vi "RT Main v0.8.vi"() -> ()   [LabVIEW 2017]
uses:
  support/Controls/All Inputs.ctl
  support/Controls/Index Details.ctl
  Controls/Auto Delays.ctl
  Global Variables/RT GV.vi
  <vilib>/Utility/error.llb/Error Cluster From Error Code.vi
  <vilib>/rvi/errors/niLvFpgaAdjustHostInterfaceError.vi
  Global Variables/FPGA GV.vi
  Global Variables/Network Globals.vi
  support/Message Queue/Enqueue Message (Single).vi
  <vilib>/FPGAPlugInAG/Dynamic/niLvFpga_Close_Dynamic.vi
  <vilib>/rvi/interface/nirviReadWriteControl/nirviReadWriteControl.xnode
  Controls/FPGA Ref.ctl
  <vilib>/rvi/interface/nirviCloseFPGA/nirviCloseFPGA.xnode
  support/Message Queue/Message Queue.lvlib
  NiFpgaLv.dll
  <vilib>/rvi/interface/Simulation/niFpgaSimulationCallBeginRW.vi
panel:
  out "BF Delays":u32[](array[numeric])=[1000, 1000]
  in  "Stop Button 3":bool
  in  "Stop Button 2":bool
  out "Agitator Delays":u32[](array[numeric])=[400, 5000]
  out "error out":errorcluster
  out "Wrong Message":string
  in  "Stop Button":bool
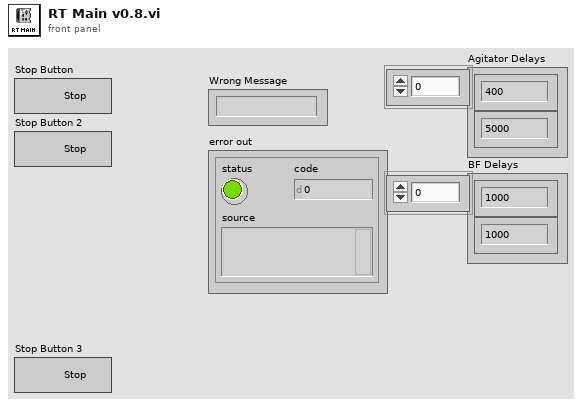
[diagram p1: front panel]
types:
  T1 = typedef "FPGA Ref.ctl" = refnum<k20>
  T2 = cluster{"TL_Red":bool, "TL_Orange":bool, "TL_Green":bool, "TL_Buzzer":bool, "SOL_Index_Rotary_CW":bool, "SOL_Index_CNVR_Rotary_CCW":bool, "SOL_Index_CNVR_Stopper_Rear":bool, "SOL_Index_CNVR_Output _Separator _Rear":bool, "Bowl  Feeder_ ON":bool, "Pump_CNVR_Motor _ON":bool, "SOL_Gating_CYL_Rear":bool, "SOL_Tube_Feed_Agitatator":bool, "SOL_Tube_Feed_Gating_CYL":bool, "SOL_Insertion _CYL":bool, "SOL_Insertion_Clamp_CYL":bool, "SOL_Cutting_CYL":bool, "SOL_Cutting_Clamp_CYL":bool, "SOL_Insertion_Air_Nozzle":bool, "SOL_Measurement_CYL":bool, "SOL_Measure_Clamp_CYL":bool, "SOL_Rejection CYL_1":bool, "SOL_Rejection CYL_2":bool, "SOL_Rejection CYL_3":bool, "SOL_Rejection CYL_4":bool, "DO1.24":bool, "DO1.25":bool, "DO1.26":bool, "DO1.27":bool, "DO1.28":bool, "DO1.29":bool, "DO1.30":bool, "DO1.31":bool}
  T3 = typedef "All Inputs.ctl" = cluster{"DI 1":cluster{"Machine_ON":bool, "E_stop ":bool, "SW_Pressure":bool, "SW_Start ":bool, "SW_Reset":bool, "SW_Stop":bool, "SW_Door":bool, "RS_Index_Rotary_CW":bool, "RS_Index_Rotary_CCW":bool, "RS_Index_Stopper _Rear":bool, "RS_Index_Output_Separator_Rear":bool, "PES_Index_Pallet_Sensor":bool, "PES_Index_Output_Part Sensor":bool, "ICS_BF_Low_Level_1":bool, "ICS_BF_Low_Level_2":bool, "ICS_BF_Pump_CNVR_Full_1":bool, "ICS_BF_Pump_CNVR_Full_2":bool, "ICS_BF_Pump_CNVR_Full_3":bool, "ICS_BF_Pump_CNVR_Full_4":bool, "PES_PC_Pump Presence_1":bool, "PES_PC_Pump Presence_2":bool, "PES_PC_Pump Presence_3":bool, "PES_PC_Pump Presence_4":bool, "RS_PC_Gating_Front":bool, "PES_Pump_Interference":bool, "PES_TF_Low_Level":bool, "PES_Tube Presence_1":bool, "PES_Tube Presence_2":bool, "PES_Tube Presence_3":bool, "PES_Tube Presence_4":bool, "DI1.30":bool, "DI1.31":bool}, "DI 2":cluster{"RS_Agitatator_1_Rear ":bool, "RS_Agitatator_2_Rear ":bool, "RS_TF_Gating CYL_Rear":bool, "RS_Insertion_1_Rear":bool, "RS_Insertion_1_Front":bool, "RS_Insertion _2_Rear":bool, "RS_Insertion _2_Front":bool, "RS_Insertion _3_Rear":bool, "RS_Insertion _3_Front":bool, "RS_Insertion _4_Rear":bool, "RS_Insertion _4_Front":bool, "RS_Insertion_Clamp_Rear":bool, "RS_Cutting_Rear":bool, "RS_Cutting_Clamp _Rear":bool, "RS_Measurement_1_Rear":bool, "RS_Measurement_2_Rear":bool, "RS_Measurement_3_Rear":bool, "RS_Measurement_4_Rear":bool, "RS_Measure_Clamp_Rear":bool, "RS_Rejection_1_Rear":bool, "RS_Rejection_2_Rear":bool, "RS_Rejection_3_Rear":bool, "RS_Rejection_4_Rear":bool, "DI2.23":bool, "DI2.24":bool, "DI2.25":bool, "DI2.26":bool, "DI2.27":bool, "DI2.28":bool, "DI2.29":bool, "DI2.30":bool, "DI2.31":bool}, "IAS 1":dbl, "IAS 2":dbl, "IAS 3":dbl, "IAS 4":dbl, "DO 1":cluster{"TL_Red":bool, "TL_Orange":bool, "TL_Green":bool, "TL_Buzzer":bool, "SOL_Index_Rotary_CW":bool, "SOL_Index_CNVR_Rotary_CCW":bool, "SOL_Index_CNVR_Stopper_Rear":bool, "SOL_Index_CNVR_Output _Separator _Rear":bool, "Bowl  Feeder_ ON 1":bool, "Pump_CNVR_Motor _ON":bool, "SOL_PC_Gating_CYL_Rear":bool, "SOL_Tube_Feed_Agitatator":bool, "SOL_Tube_Feed_Gating_CYL":bool, "SOL_Insertion _CYL":bool, "SOL_Insertion_Clamp_CYL":bool, "SOL_Cutting_CYL":bool, "SOL_Cutting_Clamp_CYL":bool, "SOL_Insertion_Air_Nozzle":bool, "SOL_Measurement_CYL":bool, "DO1.19":bool, "SOL_Rejection CYL_1":bool, "SOL_Rejection CYL_2":bool, "SOL_Rejection CYL_3":bool, "SOL_Rejection CYL_4":bool, "Bowl  Feeder_ ON 2":bool, "SOL_BF_BlowerON":bool, "SOL_BF1_Track1":bool, "SOL_BF1_Track2":bool, "SOL_BF2_Track1":bool, "SOL_BF2_Track2":bool, "DO1.30":bool, "DO1.31":bool}}
  T4 = typedef "Index Details.ctl" = cluster{"Time (ms)":u32, "Waveform Graph":i16[]}
  T5 = typedef "Auto Delays.ctl" = cluster{"Agitator Delays":u32[], "TF Delays":u32[], "Insertion Delays":u32[], "Cutting Delays":u32[], "PF Delays":u32[], "Measur. Delays":u32[], "Reject Delays":u32[], "BF Delays":u32[]}
  T6 = cluster{T5, "Reject Pallets":cluster{"Reject 1":bool, "Reject 2":bool, "Reject 3":bool, "Reject 4":bool}}
  T7 = cluster{"TL_Red":bool, "TL_Orange":bool, "TL_Green":bool, "TL_Buzzer":bool, "SOL_Index_Rotary_CW":bool, "SOL_Index_CNVR_Rotary_CCW":bool, "SOL_Index_CNVR_Stopper_Rear":bool, "SOL_Index_CNVR_Output _Separator _Rear":bool, "Bowl Feeder_ ON1":bool, "Pump_CNVR_Motor _ON":bool, "SOL_PC_Gating_CYL_Rear":bool, "SOL_Tube_Feed_Agitatator":bool, "SOL_Tube_Feed_Gating_CYL":bool, "SOL_Insertion _CYL":bool, "SOL_Insertion_Clamp_CYL":bool, "SOL_Cutting_CYL":bool, "SOL_Cutting_Clamp_CYL":bool, "SOL_Insertion_Air_Nozzle":bool, "SOL_Measurement_CYL":bool, "DO1.19":bool, "SOL_Rejection CYL_1":bool, "SOL_Rejection CYL_2":bool, "SOL_Rejection CYL_3":bool, "SOL_Rejection CYL_4":bool, "Bowl Feeder_ON2":bool, "SOL_BF_BlowerON":bool, "SOL_BF1_Track1":bool, "SOL_BF1_Track2":bool, "SOL_BF2_Track1":bool, "SOL_BF2_Track2":bool, "DO1.30":bool, "DO1.31":bool}
  T8 = cluster{"Machine_ON":bool, "E_stop ":bool, "SW_Pressure":bool, "SW_Start ":bool, "SW_Reset":bool, "SW_Stop":bool, "SW_Door":bool, "RS_Index_Rotary_CW":bool, "RS_Index_Rotary_CCW":bool, "RS_Index_Stopper _Rear":bool, "RS_Index_Output_Separator_Rear":bool, "PES_Index_Pallet_Sensor":bool, "PES_Index_Output_Part Sensor":bool, "ICS_BF_Low_Level_1":bool, "ICS_BF_Low_Level_2":bool, "ICS_BF_Pump_CNVR_Full_1":bool, "ICS_BF_Pump_CNVR_Full_2":bool, "ICS_BF_Pump_CNVR_Full_3":bool, "ICS_BF_Pump_CNVR_Full_4":bool, "PES_PC_Pump Presence_1":bool, "PES_PC_Pump Presence_2":bool, "PES_PC_Pump Presence_3":bool, "PES_PC_Pump Presence_4":bool, "RS_PC_Gating_Front":bool, "PES_Pump_Interference":bool, "PES_TF_Low_Level":bool, "PES_Tube Presence_1":bool, "PES_Tube Presence_2":bool, "PES_Tube Presence_3":bool, "PES_Tube Presence_4":bool, "DI1.30":bool, "DI1.31":bool}
  T9 = cluster{"RS_Agitatator_1_Rear ":bool, "RS_Agitatator_2_Rear ":bool, "RS_TF_Gating CYL_Rear":bool, "RS_Insertion_1_Rear":bool, "RS_Insertion_1_Front":bool, "RS_Insertion _2_Rear":bool, "RS_Insertion _2_Front":bool, "RS_Insertion _3_Rear":bool, "RS_Insertion _3_Front":bool, "RS_Insertion _4_Rear":bool, "RS_Insertion _4_Front":bool, "RS_Insertion_Clamp_Rear":bool, "RS_Cutting_Rear":bool, "RS_Cutting_Clamp _Rear":bool, "RS_Measurement_1_Rear":bool, "RS_Measurement_2_Rear":bool, "RS_Measurement_3_Rear":bool, "RS_Measurement_4_Rear":bool, "DI2.18":bool, "RS_Rejection_1_Rear":bool, "RS_Rejection_2_Rear":bool, "RS_Rejection_3_Rear":bool, "RS_Rejection_4_Rear":bool, "DI2.23":bool, "DI2.24":bool, "DI2.25":bool, "DI2.26":bool, "DI2.27":bool, "DI2.28":bool, "DI2.29":bool, "DI2.30":bool, "DI2.31":bool}
  T10 = cluster{"Reject 1":bool, "Reject 2":bool, "Reject 3":bool, "Reject 4":bool}
  T11 = typedef "Auto Times.ctl" = cluster{"Index Time":u32, "TF Time":u32, "Insertion Time":u32, "Cutting Time":u32, "PF Time":u32, "Meas. Time":u32, "Reject Time":u32}
  T12 = cluster{"Auto Times":T11, "Measurements":cluster{"1":dbl, "2":dbl, "3":dbl, "4":dbl}, "OutputCount":u32, "error out":errorcluster}
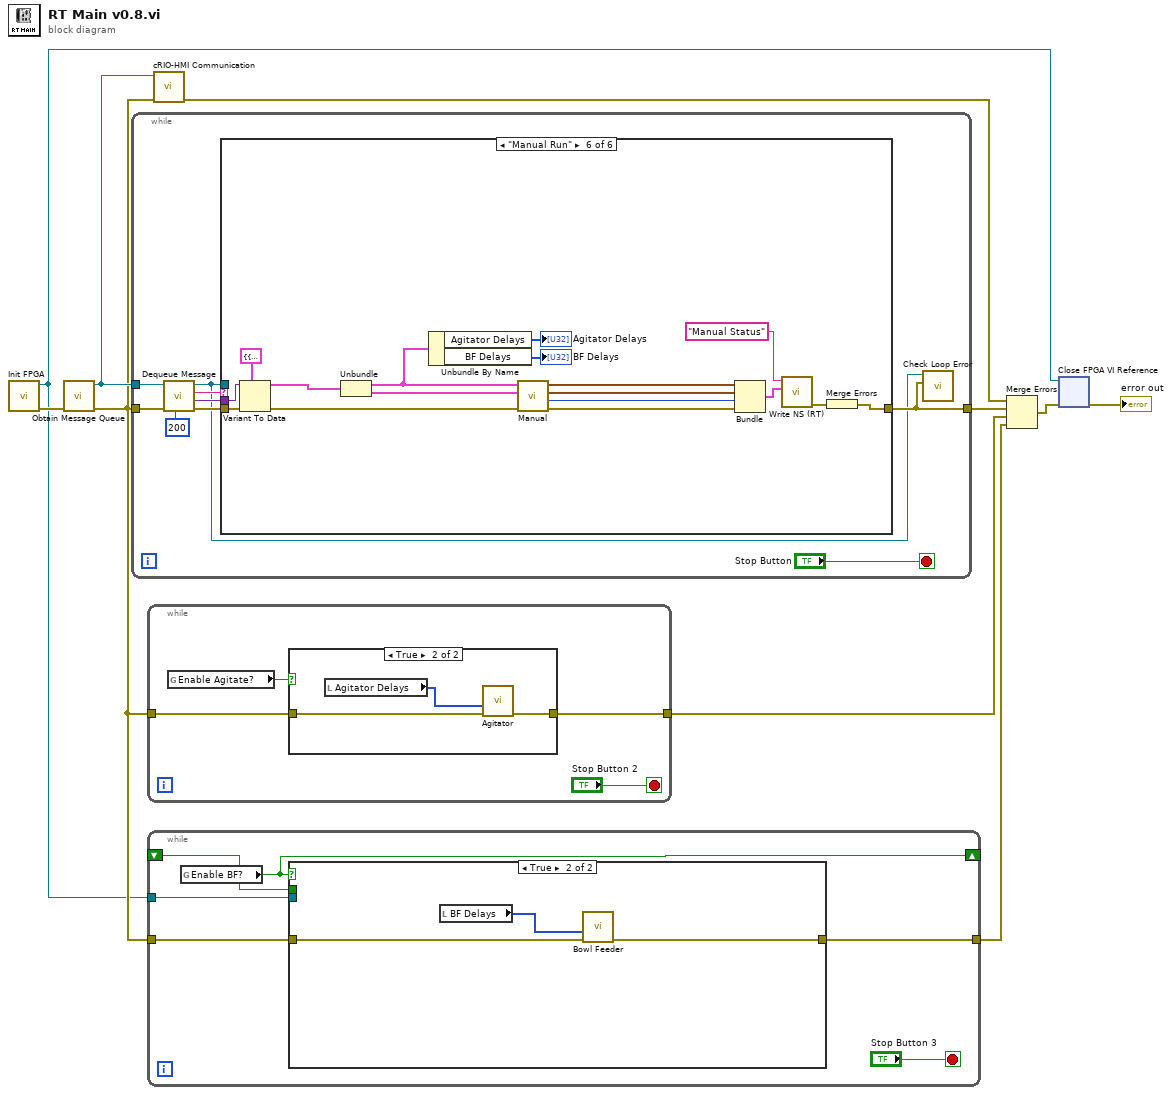
[diagram p0: block diagram]
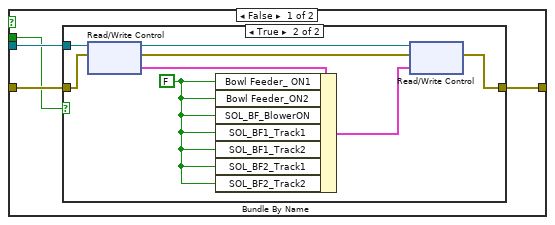
[diagram p2: hidden frame]
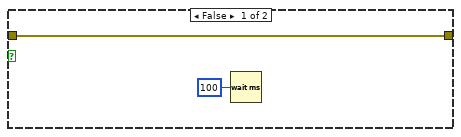
[diagram p3: hidden frame]
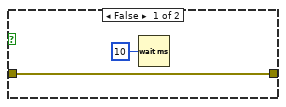
[diagram p4: hidden frame]
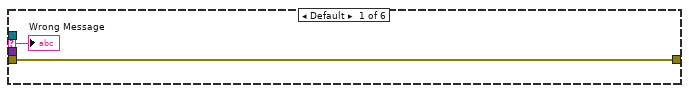
[diagram p5: hidden frame]
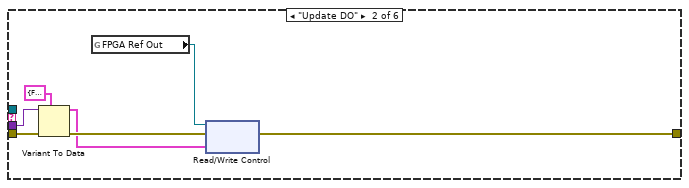
[diagram p6: hidden frame]
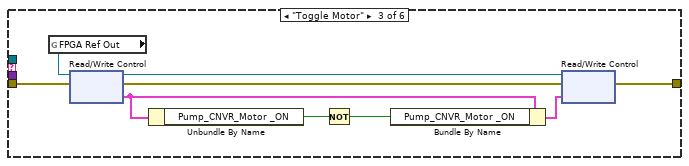
[diagram p7: hidden frame]
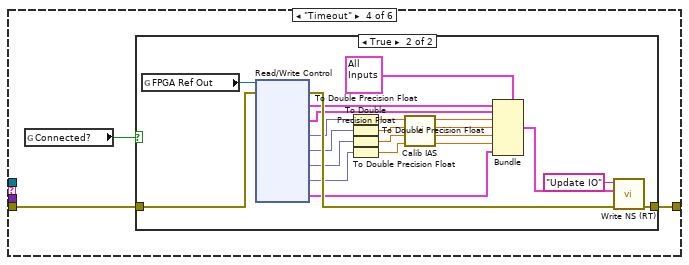
[diagram p8: hidden frame]
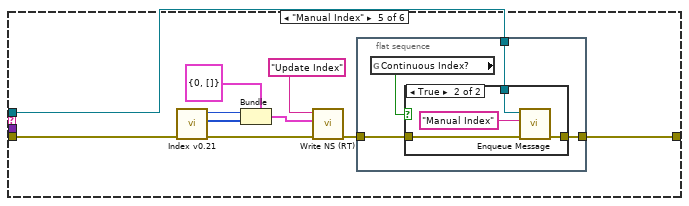
[diagram p10: hidden frame]
diagram:
  n1 = call "Init FPGA.vi"() -> ("error out"=w10:errorcluster, "FPGA Ref Out"=w1:T1)  [unwired: 10 in]
  n2 = call "Obtain Message Queue.vi"("error in (no error)"=w10) -> ("error out"=w3:errorcluster, "Message Queue"=w9:refnum<queue>)  [unwired: 9 in]
  n3 = while {
    tunnel: w3 -> [w18]
    tunnel: w9 -> [w17]
    tunnel: [w13] -> w8
    stop <- "Stop Button" stop-if-true
    n4 = call "Dequeue Message.vi"("timeout"=200, "error in (no error)"=w18, "Message Queue"=w17) -> ("error out"=w16:errorcluster, "Message Data"=w14:variant, "Message"=w15:string, "dup Message Queue"=w12:refnum<queue>)  [unwired: 5 in]
    n5 = case shown="\"Manual Run\"" w15 {
      selector: w15 -> [w21 _ _ _ _ _]
      tunnel: w16 -> [w20 w28 w36 w39 w73 w99]
      tunnel: w12 -> [_ _ _ _ w65 _]
      tunnel: w14 -> [_ w27 _ _ _ w98]
      tunnel: [w20 w23 w34 w40 w66 w94] -> w13
      frame Default {
        "Wrong Message" <- w21
      }
      frame "Update DO" {
        n6 = Variant To Data(error in=w28, type=T2 {"TL_Red"=FALSE, "TL_Orange"=FALSE, "TL_Green"=FALSE, "TL_Buzzer"=FALSE, "SOL_Index_Rotary_CW"=FALSE, "SOL_Index_CNVR_Rotary_CCW"=FALSE, "SOL_Index_CNVR_Stopper_Rear"=FALSE, "SOL_Index_CNVR_Output _Separator _Rear"=FALSE, "Bowl  Feeder_ ON"=FALSE, "Pump_CNVR_Motor _ON"=FALSE, "SOL_Gating_CYL_Rear"=FALSE, "SOL_Tube_Feed_Agitatator"=FALSE, "SOL_Tube_Feed_Gating_CYL"=FALSE, "SOL_Insertion _CYL"=FALSE, "SOL_Insertion_Clamp_CYL"=FALSE, "SOL_Cutting_CYL"=FALSE, "SOL_Cutting_Clamp_CYL"=FALSE, "SOL_Insertion_Air_Nozzle"=FALSE, "SOL_Measurement_CYL"=FALSE, "SOL_Measure_Clamp_CYL"=FALSE, "SOL_Rejection CYL_1"=FALSE, "SOL_Rejection CYL_2"=FALSE, "SOL_Rejection CYL_3"=FALSE, "SOL_Rejection CYL_4"=FALSE, "DO1.24"=FALSE, "DO1.25"=FALSE, "DO1.26"=FALSE, "DO1.27"=FALSE, "DO1.28"=FALSE, "DO1.29"=FALSE, "DO1.30"=FALSE, "DO1.31"=FALSE} ("DO 1"), Variant=w27) -> (data=w22:T2, error out=w24:errorcluster)
        n7 = global read "FPGA GV.vi" "FPGA Ref Out"() -> (w25:T1)
        n8 = xnode "Read/Write Control"("FPGA VI Reference In"=w25, "error in"=w24, "DO 1"=w22) -> ("error out"=w23:errorcluster)  [unwired: 1 out]
      }
      frame "Toggle Motor" {
        n9 = global read "FPGA GV.vi" "FPGA Ref Out"() -> (w37:T1)
        n10 = xnode "Read/Write Control"("FPGA VI Reference In"=w37, "error in"=w36) -> ("FPGA VI Reference Out"=w33:T1, "error out"=w35:errorcluster, "DO 1"=w31:T7)
        n11 = Unbundle By Name(w31) -> ("Pump_CNVR_Motor _ON"=w32:bool)
        n12 = Not(x=w32) -> (.not. x?=w29:bool)
        n13 = Bundle By Name(cluster=w31, "Pump_CNVR_Motor _ON"=w29) -> (w30:T7)
        n14 = xnode "Read/Write Control"("FPGA VI Reference In"=w33, "error in"=w35, "DO 1"=w30) -> ("error out"=w34:errorcluster)  [unwired: 1 out]
      }
      frame "Timeout" {
        n15 = global read "Network Globals.vi" "Connected?"() -> (w38:bool)
        n16 = case shown="True" w38 {
          tunnel: [w41 w62] -> w40
          tunnel: w39 -> [w41 w60]
          frame False {
          }
          frame True {
            n17 = global read "FPGA GV.vi" "FPGA Ref Out"() -> (w61:T1)
            n18 = xnode "Read/Write Control"("FPGA VI Reference In"=w61, "error in"=w60) -> ("error out"=w59:errorcluster, "DI 1"=w58:T8, "DI 2"=w57:T9, "AI0"=w56:fxp<+/-,27,6>, "AI1"=w55:fxp<+/-,27,6>, "AI2"=w54:fxp<+/-,27,6>, "AI3"=w53:fxp<+/-,27,6>, "DO 1"=w50:T7)  [unwired: 1 out]
            n19 = To Double Precision Float(number=w56) -> (double precision float=w43:dbl)
            n20 = To Double Precision Float(number=w55) -> (double precision float=w45:dbl)
            n21 = To Double Precision Float(number=w54) -> (double precision float=w47:dbl)
            n22 = To Double Precision Float(number=w53) -> (double precision float=w49:dbl)
            n23 = call "Calib IAS.vi"("x 4"=w49, "x 3"=w47, "x 2"=w45, "x"=w43) -> ("y 4"=w48:dbl, "y 3"=w46:dbl, "y 2"=w44:dbl, "y 1"=w42:dbl)  [unwired: 4 in]
            n24 = Bundle(cluster=T3 {"DI 1"={"Machine_ON"=FALSE, "E_stop "=FALSE, "SW_Pressure"=FALSE, "SW_Start "=FALSE, "SW_Reset"=FALSE, "SW_Stop"=FALSE, "SW_Door"=FALSE, "RS_Index_Rotary_CW"=FALSE, "RS_Index_Rotary_CCW"=FALSE, "RS_Index_Stopper _Rear"=FALSE, "RS_Index_Output_Separator_Rear"=FALSE, "PES_Index_Pallet_Sensor"=FALSE, "PES_Index_Output_Part Sensor"=FALSE, "ICS_BF_Low_Level_1"=FALSE, "ICS_BF_Low_Level_2"=FALSE, "ICS_BF_Pump_CNVR_Full_1"=FALSE, "ICS_BF_Pump_CNVR_Full_2"=FALSE, "ICS_BF_Pump_CNVR_Full_3"=FALSE, "ICS_BF_Pump_CNVR_Full_4"=FALSE, "PES_PC_Pump Presence_1"=FALSE, "PES_PC_Pump Presence_2"=FALSE, "PES_PC_Pump Presence_3"=FALSE, "PES_PC_Pump Presence_4"=FALSE, "RS_PC_Gating_Front"=FALSE, "PES_Pump_Interference"=FALSE, "PES_TF_Low_Level"=FALSE, "PES_Tube Presence_1"=FALSE, "PES_Tube Presence_2"=FALSE, "PES_Tube Presence_3"=FALSE, "PES_Tube Presence_4"=FALSE, "DI1.30"=FALSE, "DI1.31"=FALSE}, "DI 2"={"RS_Agitatator_1_Rear "=FALSE, "RS_Agitatator_2_Rear "=FALSE, "RS_TF_Gating CYL_Rear"=FALSE, "RS_Insertion_1_Rear"=FALSE, "RS_Insertion_1_Front"=FALSE, "RS_Insertion _2_Rear"=FALSE, "RS_Insertion _2_Front"=FALSE, "RS_Insertion _3_Rear"=FALSE, "RS_Insertion _3_Front"=FALSE, "RS_Insertion _4_Rear"=FALSE, "RS_Insertion _4_Front"=FALSE, "RS_Insertion_Clamp_Rear"=FALSE, "RS_Cutting_Rear"=FALSE, "RS_Cutting_Clamp _Rear"=FALSE, "RS_Measurement_1_Rear"=FALSE, "RS_Measurement_2_Rear"=FALSE, "RS_Measurement_3_Rear"=FALSE, "RS_Measurement_4_Rear"=FALSE, "RS_Measure_Clamp_Rear"=FALSE, "RS_Rejection_1_Rear"=FALSE, "RS_Rejection_2_Rear"=FALSE, "RS_Rejection_3_Rear"=FALSE, "RS_Rejection_4_Rear"=FALSE, "DI2.23"=FALSE, "DI2.24"=FALSE, "DI2.25"=FALSE, "DI2.26"=FALSE, "DI2.27"=FALSE, "DI2.28"=FALSE, "DI2.29"=FALSE, "DI2.30"=FALSE, "DI2.31"=FALSE}, "IAS 1"=0.0, "IAS 2"=0.0, "IAS 3"=0.0, "IAS 4"=0.0, "DO 1"={"TL_Red"=FALSE, "TL_Orange"=FALSE, "TL_Green"=FALSE, "TL_Buzzer"=FALSE, "SOL_Index_Rotary_CW"=FALSE, "SOL_Index_CNVR_Rotary_CCW"=FALSE, "SOL_Index_CNVR_Stopper_Rear"=FALSE, "SOL_Index_CNVR_Output _Separator _Rear"=FALSE, "Bowl  Feeder_ ON 1"=FALSE, "Pump_CNVR_Motor _ON"=FALSE, "SOL_PC_Gating_CYL_Rear"=FALSE, "SOL_Tube_Feed_Agitatator"=FALSE, "SOL_Tube_Feed_Gating_CYL"=FALSE, "SOL_Insertion _CYL"=FALSE, "SOL_Insertion_Clamp_CYL"=FALSE, "SOL_Cutting_CYL"=FALSE, "SOL_Cutting_Clamp_CYL"=FALSE, "SOL_Insertion_Air_Nozzle"=FALSE, "SOL_Measurement_CYL"=FALSE, "DO1.19"=FALSE, "SOL_Rejection CYL_1"=FALSE, "SOL_Rejection CYL_2"=FALSE, "SOL_Rejection CYL_3"=FALSE, "SOL_Rejection CYL_4"=FALSE, "Bowl  Feeder_ ON 2"=FALSE, "SOL_BF_BlowerON"=FALSE, "SOL_BF1_Track1"=FALSE, "SOL_BF1_Track2"=FALSE, "SOL_BF2_Track1"=FALSE, "SOL_BF2_Track2"=FALSE, "DO1.30"=FALSE, "DO1.31"=FALSE}}, "DI 1"=w58, "DI 2"=w57, "IAS 1"=w42, "IAS 2"=w44, "IAS 3"=w46, "IAS 4"=w48, "DO 1"=w50) -> (w52:T3)
            n25 = call "Write NS (RT).vi"("error in (no error)"=w59, "Message Data"=w52, "Message"="Update IO") -> ("error out"=w62:errorcluster)  [unwired: 8 in]
          }
        }
      }
      frame "Manual Index" {
        n26 = call "Index v0.21.vi"("error in (no error)"=w73) -> ("error out"=w71:errorcluster, "Waveform Graph"=w69:i16[], "Index Time"=w70:u32)  [unwired: 7 in, 1 out]
        n27 = Bundle(cluster=T4 {"Time (ms)"=0, "Waveform Graph"=[]}, "Time (ms)"=w70, "Waveform Graph"=w69) -> (w68:T4)
        n28 = call "Write NS (RT).vi"("error in (no error)"=w71, "Message Data"=w68, "Message"="Update Index") -> ("error out"=w67:errorcluster)  [unwired: 8 in]
        n29 = flat-sequence {
          tunnel: w67 -> [w77]
          tunnel: [w76] -> w66
          tunnel: w65 -> [w74]
          frame #0 {
            n30 = global read "RT GV.vi" "Continuous Index?"() -> (w75:bool)
            n31 = case shown="True" w75 {
              tunnel: w77 -> [w78 w82]
              tunnel: [w78 w81] -> w76
              tunnel: w74 -> [_ w79]
              frame False {
              }
              frame True {
                n32 = call-poly "Enqueue Message.vi"("error in (no error)"=w82, "Message"="Manual Index", "Message Queue"=w79) -> ("error out"=w81:errorcluster)  [unwired: 7 in, 1 out]
              }
            }
          }
        }
      }
      frame "Manual Run" {
        n33 = Variant To Data(error in=w99, type=T6 {{"Agitator Delays"=[1000], "TF Delays"=[1000], "Insertion Delays"=[1000], "Cutting Delays"=[1000], "PF Delays"=[1000], "Measur. Delays"=[1000], "Reject Delays"=[1000], "BF Delays"=[1000]}, "Reject Pallets"={"Reject 1"=FALSE, "Reject 2"=FALSE, "Reject 3"=FALSE, "Reject 4"=FALSE}}, Variant=w98) -> (data=w89:T6, error out=w97:errorcluster)
        n34 = Unbundle(w89) -> (w85:T5, "Reject Pallets"=w88:T10)
        n35 = Unbundle By Name(w85) -> ("Agitator Delays"=→"Agitator Delays":u32[], "BF Delays"=→"BF Delays":u32[])
        n36 = call "Manual.vi"("error in (no error)"=w97, "Reject Pallets"=w88, "Auto Delays"=w85) -> ("error out"=w87:errorcluster, "OutputCount"=w86:u32, "Measurements"=w91:cluster{"1":dbl, "2":dbl, "3":dbl, "4":dbl}, "Auto Times"=w93:T11)  [unwired: 5 in]
        n37 = Bundle("Auto Times"=w93, "Measurements"=w91, "OutputCount"=w86, "error out"=w87) -> (w92:T12)  [unwired: 1 in]
        n38 = call "Write NS (RT).vi"("Message Data"=w92, "Message"="Manual Status") -> ("error out"=w95:errorcluster)  [unwired: 9 in]
        n39 = Merge Errors(w95) -> (w94:errorcluster)
      }
    }
    n40 = call "Check Loop Error.vi"("error to process"=w13, "Message Queue"=w12) -> ()  [unwired: 8 in, 2 out]
  }
  n41 = while {
    tunnel: w3 -> [w103]
    tunnel: [w100] -> w4
    stop <- "Stop Button 2" stop-if-true
    n42 = global read "RT GV.vi" "Enable Agitate?"() -> (w102:bool)
    n43 = case shown="True" w102 {
      tunnel: w103 -> [w105 w108]
      tunnel: [w105 w106] -> w100
      frame False {
        n44 = Wait (ms)(milliseconds to wait=u32 10) -> ()  [unwired: 1 out]
      }
      frame True {
        n45 = local read "Agitator Delays"() -> (w107:u32[])
        n46 = call "Agitator.vi"("error in (no error)"=w108, "Agitator Delays"=w107) -> ("error out"=w106:errorcluster)  [unwired: 8 in, 1 out]
      }
    }
  }
  n47 = while {
    tunnel: w3 -> [w114]
    tunnel: [w112] -> w2
    shift-right: [w111] -> _
    shift-left: _ -> [w110]
    tunnel: w1 -> [w109]
    stop <- "Stop Button 3" stop-if-true
    n48 = global read "RT GV.vi" "Enable BF?"() -> (w111:bool)
    n49 = case shown="True" w111 {
      tunnel: w114 -> [w118 w131]
      tunnel: [w117 w129] -> w112
      tunnel: w110 -> [w115 _]
      tunnel: w109 -> [w116 _]
      frame False {
        n50 = case shown="True" w115 {
          tunnel: w118 -> [w119 w123]
          tunnel: [w119 w122] -> w117
          tunnel: w116 -> [_ w121]
          frame False {
            n51 = Wait (ms)(milliseconds to wait=u32 100) -> ()  [unwired: 1 out]
          }
          frame True {
            w124 = FALSE ("SOL_Index_Rotary_CW")
            n52 = xnode "Read/Write Control"("FPGA VI Reference In"=w121, "error in"=w123) -> ("FPGA VI Reference Out"=w125:T1, "error out"=w126:errorcluster, "DO 1"=w127:T7)
            n53 = Bundle By Name(cluster=w127, "Bowl Feeder_ ON1"=w124, "Bowl Feeder_ON2"=w124, "SOL_BF_BlowerON"=w124, "SOL_BF1_Track1"=w124, "SOL_BF1_Track2"=w124, "SOL_BF2_Track1"=w124, "SOL_BF2_Track2"=w124) -> (w128:T7)
            n54 = xnode "Read/Write Control"("FPGA VI Reference In"=w125, "error in"=w126, "DO 1"=w128) -> ("error out"=w122:errorcluster)  [unwired: 1 out]
          }
        }
      }
      frame True {
        n55 = local read "BF Delays"() -> (w130:u32[])
        n56 = call "Bowl Feeder.vi"("error in (no error)"=w131, "BF Delays"=w130) -> ("error out"=w129:errorcluster)  [unwired: 8 in, 1 out]
      }
    }
  }
  n57 = call "cRIO-HMI Communication.vi"("error in (no error)"=w3, "Message Queue"=w9) -> ("error out"=w7:errorcluster)  [unwired: 9 in]
  n58 = Merge Errors(w7, w8, w4, w2) -> (w6:errorcluster)
  n59 = xnode ("Close FPGA VI Reference")("FPGA VI Reference In"=w1, "error in"=w6) -> ("error out"=→"error out":errorcluster)
